vi "MonoScan.vi"() -> (3 "Cancelled?":bool)   [LabVIEW 2017]
doc: "Use this template to create a dialog box. This template polls the state of the buttons on the front panel and does not use events. Use the Dialog Using Events template (not available in Base package) to create a dialog box with event handling."
panel:
  in  "Boolean 4":bool
  in  "error in (no error)":errorcluster
  out "error out":errorcluster
  in  "Delay(ms)":u32=10
  out "# of Bytes Read":u32=50
  out "error out 2":errorcluster
  out "String Read 2":string
  out "String Read":string
  in  "String":string
  in  "OK Button 3":bool
  in  "OK Button 2":bool
  in  "OK Button":bool
  in  "error in (no error) 4":errorcluster
  out "error out 8":errorcluster
  in  "Delay(ms) 4":u32=10
  in  "OK Button 8":bool
  in  "error in (no error) 2":errorcluster
  out "error out 3":errorcluster
  in  "Delay(ms) 2":u32=10
  out "Mono":string
  out "String 6":string
  out "String 5":string
  out "String 2":string
  out "String 3":string
  out "String 4":string
  out "String 7":string
  out "error out 4":errorcluster
  out "# of Bytes Read 2":u32=50
  in  "error in (no error) 3":errorcluster
  out "error out 5":errorcluster
  in  "Delay(ms) 3":u32=10
  out "error out 6":errorcluster
  out "# of Bytes Read 3":u32=50
  out "Boolean":bool
  out "Boolean 2":bool
  out "Boolean 3":bool
  in  "Port":i32
  in  "Cancel":bool
  in  "OK":bool
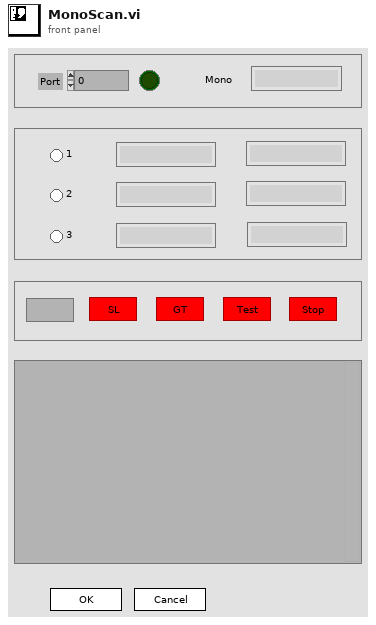
[diagram p1: front panel]
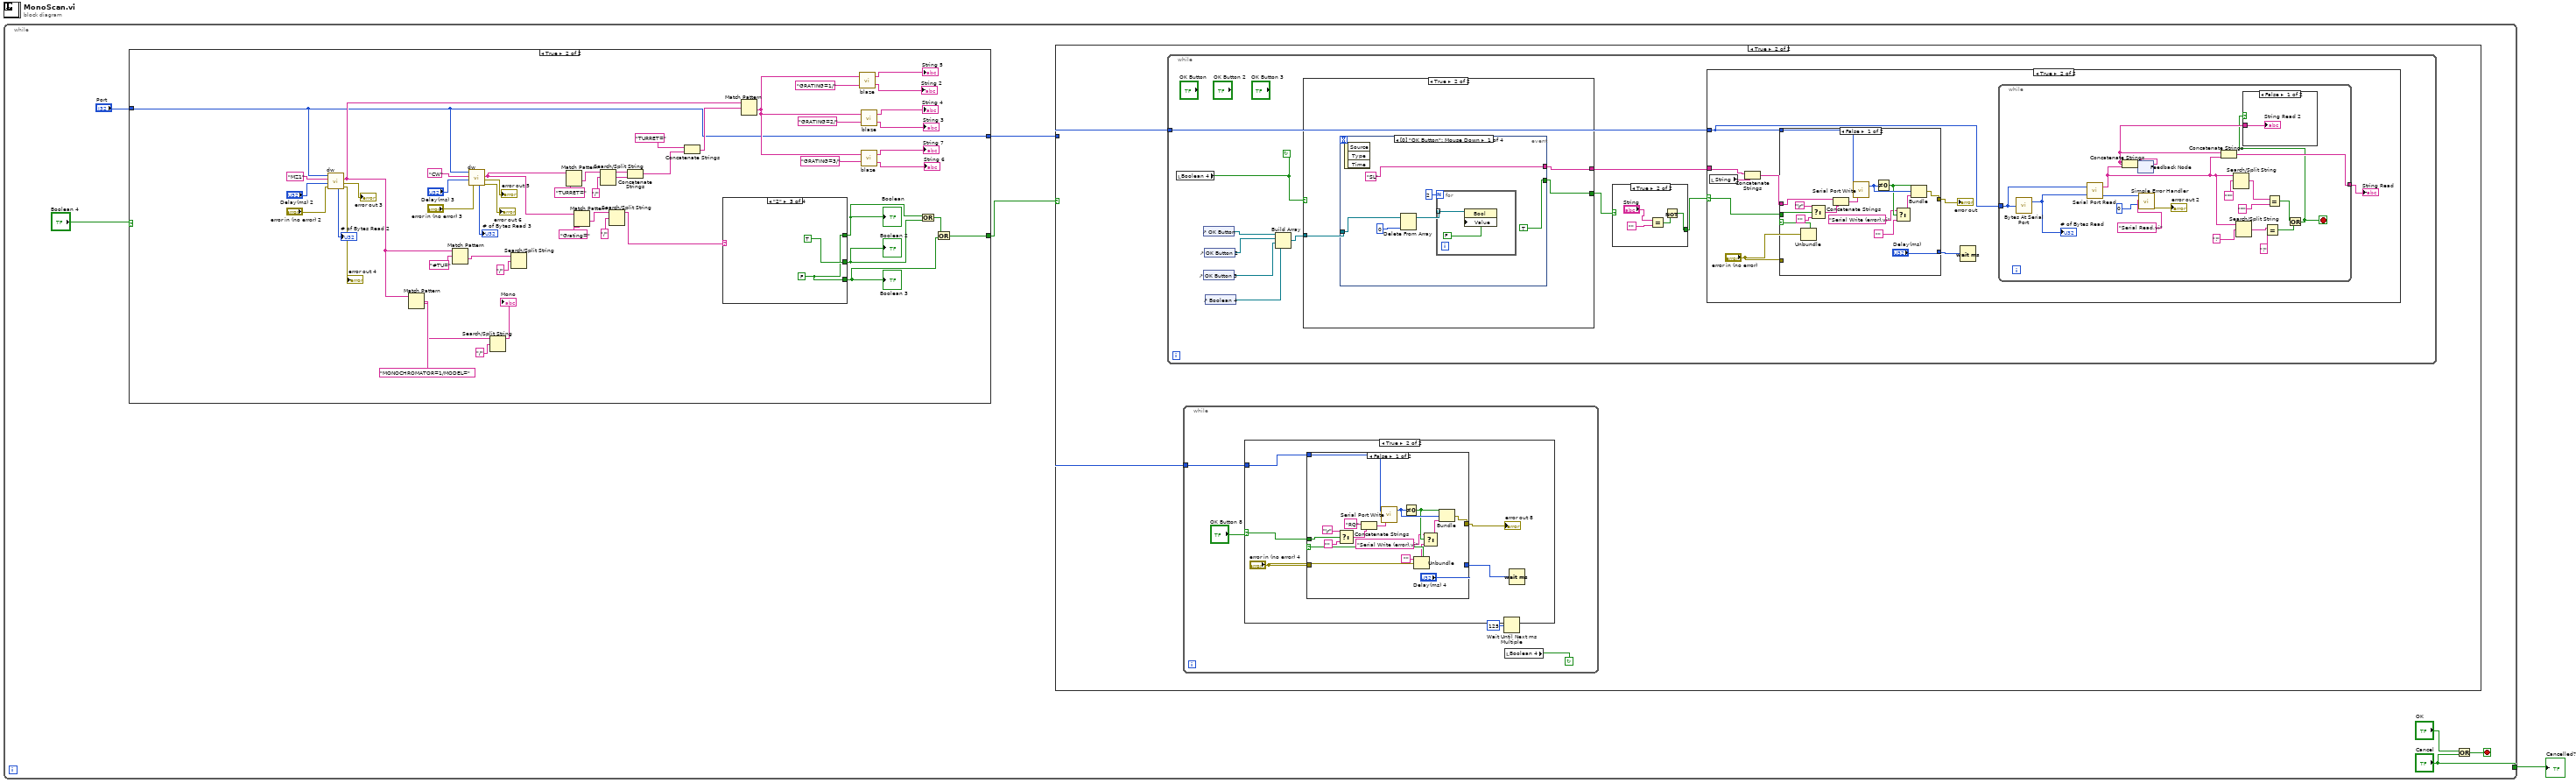
[diagram p0: block diagram]
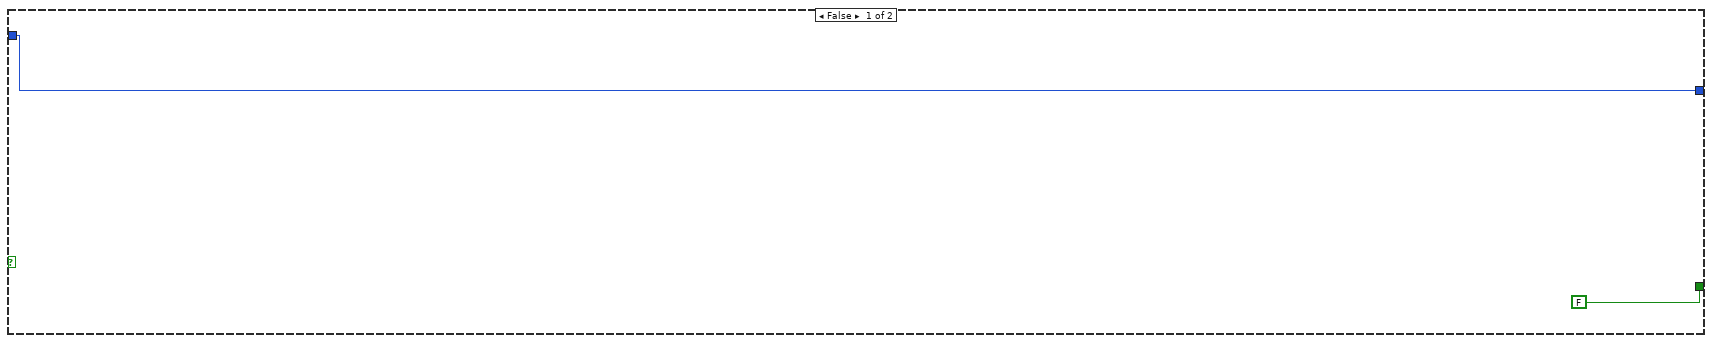
[diagram p2: hidden frame]
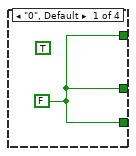
[diagram p3: hidden frame]
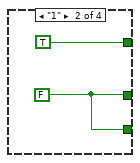
[diagram p4: hidden frame]
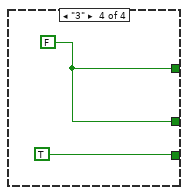
[diagram p5: hidden frame]
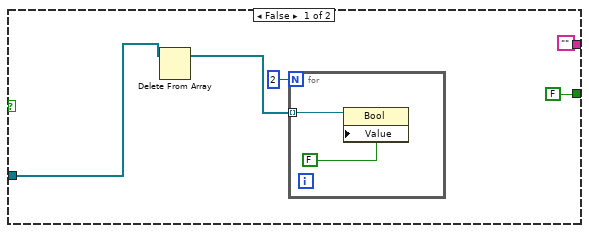
[diagram p10: hidden frame]
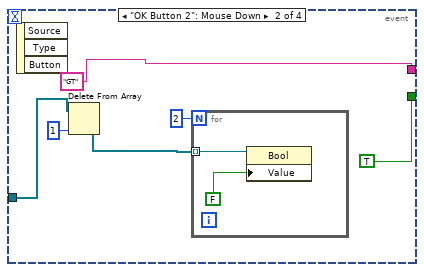
[diagram p11: hidden frame]
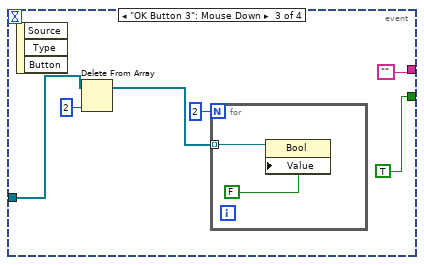
[diagram p12: hidden frame]
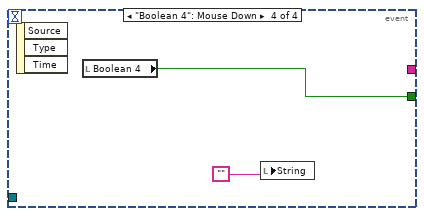
[diagram p13: hidden frame]
diagram:
  n1 = while {
    tunnel: ["Cancel"] -> w1
    stop <- w8 stop-if-true
    n2 = case shown="True" "Boolean 4" {
      tunnel: [FALSE w14] -> w5
      tunnel: [w10 w13] -> w4
      tunnel: "Port" -> [w10 w13]
      frame False {
      }
      frame True {
        n3 = call "dw.vi"("Port"=w13, "String 2"="MZ1", "Delay(ms)"="Delay(ms) 2", "error in (no error)"="error in (no error) 2") -> ("# of Bytes Read"=→"# of Bytes Read 2":u32, "String"=w50:string, "error out"=→"error out 3":errorcluster, "error out 2"=→"error out 4":errorcluster)  [unwired: 1 out]
        n4 = Match Pattern(string=w50, regular expression="MONOCHROMATOR=1/MODEL=" ("search string")) -> (after substring=w56:string)  [unwired: 1 in, 3 out]
        n5 = Match Pattern(string=w50, regular expression="#TU=") -> (after substring=w53:string)  [unwired: 1 in, 3 out]
        n6 = call "dw.vi"("Port"=w13, "String 2"="CW", "Delay(ms)"="Delay(ms) 3", "error in (no error)"="error in (no error) 3") -> ("# of Bytes Read"=→"# of Bytes Read 3":u32, "String"=w20:string, "error out"=→"error out 5":errorcluster, "error out 2"=→"error out 6":errorcluster)  [unwired: 1 out]
        n7 = Search/Split String(string=w56, search string/char (-)="/") -> (substring before match=→"Mono":string)  [unwired: 1 in, 2 out]
        n8 = Search/Split String(string=w53, search string/char (-)="/") -> ()  [unwired: 1 in, 3 out]
        n9 = Match Pattern(string=w20, regular expression="TURRET=") -> (after substring=w29:string)  [unwired: 1 in, 3 out]
        n10 = Match Pattern(string=w20, regular expression="Grating=") -> (after substring=w21:string)  [unwired: 1 in, 3 out]
        n11 = Search/Split String(string=w29, search string/char (-)="/") -> (substring before match=w25:string, match + rest of string=w26:string)  [unwired: 1 in, 1 out]
        n12 = Search/Split String(string=w21, search string/char (-)="/") -> (substring before match=w19:string)  [unwired: 1 in, 2 out]
        n13 = Concatenate Strings(w25, w26) -> (w24:string)
        n14 = Concatenate Strings("TURRET=" ("regular expression"), w24) -> (w28:string)
        n15 = case shown="\"2\"" w19 {
          tunnel: [w61 TRUE w64 w66] -> w18
          tunnel: [w61 w62 TRUE w66] -> w17
          tunnel: [w61 w62 w64 TRUE] -> w15
          frame "0", Default {
            w61 = FALSE
            (unwired) TRUE
          }
          frame "1" {
            w62 = FALSE
          }
          frame "2" {
            w64 = FALSE
          }
          frame "3" {
            w66 = FALSE
          }
        }
        "Boolean" <- w18
        "Boolean 2" <- w17
        "Boolean 3" <- w15
        n16 = Match Pattern(string=w50, regular expression=w28) -> (after substring=w43:string)  [unwired: 1 in, 3 out]
        n17 = call "blaze.vi"("String 2"="GRATING=1/", "String"=w43) -> ("String 5"=→"String 2":string, "String 4"=→"String 5":string)
        n18 = call "blaze.vi"("String 2"="GRATING=3/", "String"=w43) -> ("String 5"=→"String 6":string, "String 4"=→"String 7":string)
        n19 = call "blaze.vi"("String 2"="GRATING=2/", "String"=w43) -> ("String 5"=→"String 3":string, "String 4"=→"String 4":string)
        n20 = Or(x=w18, y=w17) -> (x .or. y?=w16:bool)
        n21 = Or(x=w16, y=w15) -> (x .or. y?=w14:bool)
      }
    }
    n22 = case shown="True" w5 {
      tunnel: w4 -> [_ w68]
      frame False {
      }
      frame True {
        n23 = while {
          tunnel: w68 -> [w103]
          stop <- w97 continue-if-true
          n24 = local read "Boolean 4"() -> (w97:bool)
          n25 = control-ref of="OK Button 3"() -> (w100:refnum<vi>)
          n26 = control-ref of="OK Button"() -> (w102:refnum<vi>)
          n27 = control-ref of="OK Button 2"() -> (w101:refnum<vi>)
          n28 = control-ref of="Boolean 4"() -> (w98:refnum<vi>)
          n29 = Build Array(w102, w101, w100, w98) -> (w99:refnum<vi>[])
          n30 = case shown="True" w97 {
            tunnel: ["" w118] -> w94
            tunnel: [FALSE w117] -> w96
            tunnel: w99 -> [w111 w116]
            frame False {
              n31 = Delete From Array(array=w111) -> (array with subset deleted=w113:refnum<vi>[])  [unwired: 2 in, 1 out]
              n32 = for {
                N: 2 -> [_]
                tunnel: w113 -> [w114] mode=indexing
                n33 = property class="Bool"(reference=w114, "Value"=FALSE) -> ()  [unwired: 1 in, 2 out]
              }
            }
            frame True {
              n34 = event shown="[0] \"OK Button\": Mouse Down" {
                selector: _ -> [_ _ _ _]
                dyn-events: _ -> [_ _ _ _]
                timeout: _ -> [_ _ _ _]
                tunnel: ["SL" "GT" "" _] -> w118
                tunnel: w116 -> [w123 w131 w139 _]
                tunnel: [TRUE TRUE TRUE w144] -> w117
                event "OK Button": Mouse Down {
                  n35 = event-data() -> ()  [unwired: 1 in, 3 out]
                  n36 = Delete From Array(array=w123, index=0) -> (array with subset deleted=w122:refnum<vi>[])  [unwired: 1 in, 1 out]
                  n37 = for {
                    N: 2 -> [_]
                    tunnel: w122 -> [w125] mode=indexing
                    n38 = property class="Bool"(reference=w125, "Value"=FALSE) -> ()  [unwired: 1 in, 2 out]
                  }
                }
                event "OK Button 2": Mouse Down {
                  n39 = event-data() -> ()  [unwired: 1 in, 3 out]
                  n40 = Delete From Array(array=w131, index=1) -> (array with subset deleted=w130:refnum<vi>[])  [unwired: 1 in, 1 out]
                  n41 = for {
                    N: 2 -> [_]
                    tunnel: w130 -> [w133] mode=indexing
                    n42 = property class="Bool"(reference=w133, "Value"=FALSE) -> ()  [unwired: 1 in, 2 out]
                  }
                }
                event "OK Button 3": Mouse Down {
                  n43 = event-data() -> ()  [unwired: 1 in, 3 out]
                  n44 = Delete From Array(array=w139, index=2) -> (array with subset deleted=w138:refnum<vi>[])  [unwired: 1 in, 1 out]
                  n45 = for {
                    N: 2 -> [_]
                    tunnel: w138 -> [w141] mode=indexing
                    n46 = property class="Bool"(reference=w141, "Value"=FALSE) -> ()  [unwired: 1 in, 2 out]
                  }
                }
                event "Boolean 4": Mouse Down {
                  n47 = event-data() -> ()  [unwired: 1 in, 3 out]
                  n48 = local read "Boolean 4"() -> (w144:bool)
                  n49 = local write "String"("") -> ()
                }
              }
            }
          }
          n50 = case shown="True" w96 {
            selector: w96 -> [w104 _]
            tunnel: [w104 w105] -> w95
            frame False {
            }
            frame True {
              n51 = Equal?(x="String", y="") -> (x = y?=w106:bool)
              n52 = Not(x=w106) -> (.not. x?=w105:bool)
            }
          }
          n53 = case shown="True" w95 {
            selector: w95 -> [_ w147]
            tunnel: w94 -> [_ w149]
            tunnel: w103 -> [_ w146]
            frame False {
            }
            frame True {
              n54 = local read "String"() -> (w145:string)
              n55 = Concatenate Strings(w149, w145) -> (w148:string)
              n56 = Unbundle("error in (no error)") -> ("status"=w153:bool)  [unwired: 2 out]
              n57 = case shown="False" w153 {
                tunnel: "error in (no error)" -> [_ w189]
                tunnel: [w184 w189] -> w152
                tunnel: w148 -> [w187 _]
                tunnel: ["Delay(ms)" 0] -> w151
                tunnel: w147 -> [w177 _]
                tunnel: w146 -> [w175 _]
                frame False {
                  n58 = Select(t="\r", s=w177, f="") -> (s? t:f=w182:string)
                  n59 = Concatenate Strings(w187, w182) -> (w186:string)
                  n60 = call <vilib>:"Serial Port Write.vi"("string to write"=w186, "port number"=w175) -> ("error code"=w185:i32)
                  n61 = Not Equal To 0?(x=w185) -> (x != 0?=w181:bool)
                  n62 = Select(t="Serial Write (error).vi", s=w181, f="") -> (s? t:f=w178:string)
                  n63 = Bundle(w181, "error code"=w185, w178) -> (w184:cluster{bool, "error code":i32, string})  [unwired: 1 in]
                }
                frame True {
                }
              }
              "error out" <- w152
              n64 = Wait (ms)(milliseconds to wait=w151) -> ()  [unwired: 1 out]
              n65 = while {
                tunnel: [w165] -> w150
                tunnel: w146 -> [w156]
                stop <- w155 stop-if-true
                n66 = call <vilib>:"Bytes At Serial Port.vi"("port number"=w156) -> ("byte count"=w170:u32)  [unwired: 1 out]
                "# of Bytes Read" <- w170
                n67 = call <vilib>:"Serial Port Read.vi"("requested byte count"=w170, "port number"=w156) -> ("error code"=w173:i32, "string read"=w163:string)
                n68 = feedback #1() -> (w157:string)  [unwired: 1 in]
                n69 = Concatenate Strings(w157, w163) -> (w167:string)
                n70 = feedback-in #1(w167) -> ()
                n71 = call <vilib>:"Simple Error Handler.vi"("error code (no error:0)"=w173, "error source (\" \")"="Serial Read.vi", "type of dialog (OK msg:1)"=0) -> ("error out"=→"error out 2":errorcluster)  [unwired: 2 in, 4 out]
                n72 = Concatenate Strings(w157, w163) -> (w165:string)
                n73 = Search/Split String(string=w163, search string/char (-)="*") -> (match + rest of string=w166:string)  [unwired: 1 in, 2 out]
                n74 = Search/Split String(string=w163, search string/char (-)="!") -> (match + rest of string=w161:string)  [unwired: 1 in, 2 out]
                n75 = Equal?(x=w161, y="!") -> (x = y?=w158:bool)
                n76 = Equal?(x=w166, y="*") -> (x = y?=w159:bool)
                n77 = Or(x=w159, y=w158) -> (x .or. y?=w155:bool)
                n78 = case shown="False" w155 {
                  tunnel: w157 -> [w174 _]
                  frame False {
                    "String Read 2" <- w174
                  }
                  frame True {
                  }
                }
              }
              "String Read" <- w150
            }
          }
        }
        n79 = while {
          tunnel: w68 -> [w70]
          stop <- w69 continue-if-true
          n80 = case shown="True" "OK Button 8" {
            selector: "OK Button 8" -> [_ w73]
            tunnel: w70 -> [_ w72]
            frame False {
            }
            frame True {
              n81 = Unbundle("error in (no error) 4") -> ("status"=w76:bool)  [unwired: 2 out]
              n82 = case shown="False" w76 {
                tunnel: "error in (no error) 4" -> [_ w92]
                tunnel: [w88 w92] -> w75
                tunnel: ["Delay(ms) 4" 0] -> w74
                tunnel: w73 -> [w81 _]
                tunnel: w72 -> [w79 _]
                frame False {
                  n83 = Select(t="\r", s=w81, f="") -> (s? t:f=w86:string)
                  n84 = Concatenate Strings("RQ" ("string"), w86) -> (w90:string)
                  n85 = call <vilib>:"Serial Port Write.vi"("string to write"=w90, "port number"=w79) -> ("error code"=w89:i32)
                  n86 = Not Equal To 0?(x=w89) -> (x != 0?=w85:bool)
                  n87 = Select(t="Serial Write (error).vi", s=w85, f="") -> (s? t:f=w82:string)
                  n88 = Bundle(w85, "error code"=w89, w82) -> (w88:cluster{bool, "error code":i32, string})  [unwired: 1 in]
                }
                frame True {
                }
              }
              "error out 8" <- w75
              n89 = Wait (ms)(milliseconds to wait=w74) -> ()  [unwired: 1 out]
            }
          }
          n90 = local read "Boolean 4"() -> (w69:bool)
        }
      }
    }
    n91 = Wait Until Next ms Multiple(millisecond multiple=u32 125) -> ()  [unwired: 1 out]
    n92 = Or(x="OK", y="Cancel") -> (x .or. y?=w8:bool)
  }
  "Cancelled?" <- w1
